vi "L Arm Initial Position.vi"(0 "Cluster":T1={"Axis"={"X"=0.0, "Y"=0.0, "Z"=0.0}, "Arm"=refnum, "EJC"=refnum, "Shoulder Angle"=0.0, "Shoulder Axis"={"X"=-1.0, "Y"=0.0, "Z"=0.0}, "Elbow Angle"=0.0, "Elbow Axis"={"X"=0.0, "Y"=-1.0, "Z"=0.0}}) -> (1 "Scene.Object Out":refnum<vi>, 3 "Scene.Object Out 3":refnum<vi>)   [LabVIEW 2010]
uses:
  <vilib>/picture/3D Picture Control/NI_3D Picture Control.lvlib
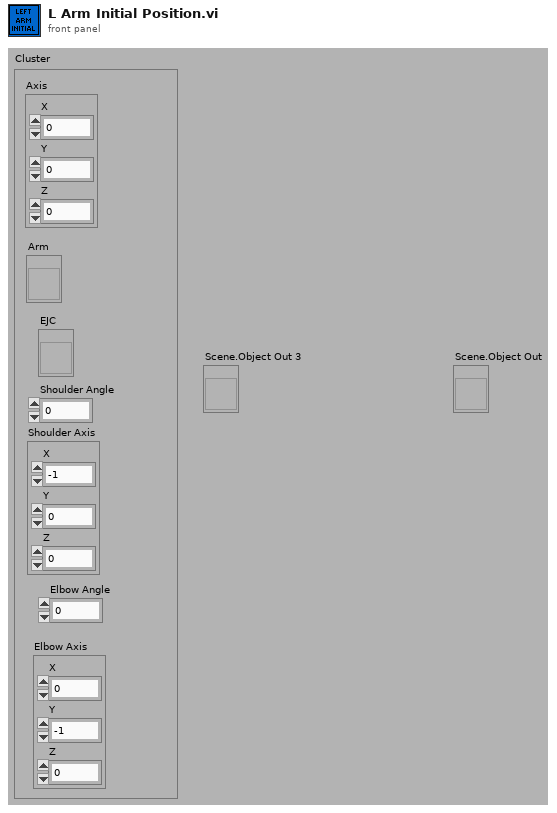
[diagram p1: front panel]
types:
  T1 = cluster{"Axis":cluster{"X":sgl, "Y":sgl, "Z":sgl}, "Arm":refnum<vi>, "EJC":refnum<vi>, "Shoulder Angle":dbl, "Shoulder Axis":cluster{"X":sgl, "Y":sgl, "Z":sgl}, "Elbow Angle":dbl, "Elbow Axis":cluster{"X":sgl, "Y":sgl, "Z":sgl}}
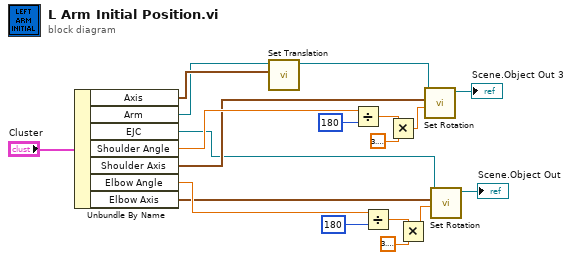
[diagram p0: block diagram]
diagram:
  n1 = Unbundle By Name("Cluster") -> ("Axis"=w4:cluster{"X":sgl, "Y":sgl, "Z":sgl}, "Arm"=w3:refnum<vi>, "EJC"=w2:refnum<vi>, "Shoulder Angle"=w8:dbl, "Shoulder Axis"=w7:cluster{"X":sgl, "Y":sgl, "Z":sgl}, "Elbow Angle"=w6:dbl, "Elbow Axis"=w5:cluster{"X":sgl, "Y":sgl, "Z":sgl})
  n2 = call <vilib>:"Set Translation.vi"("Translation"=w4, "Scene Object"=w3) -> ("Translated Object"=w1:refnum<vi>)  [unwired: 8 in, 1 out]
  n3 = Divide(x=w8, y=180) -> (x/y=w16:dbl)
  n4 = Divide(x=w6, y=180) -> (x/y=w11:dbl)
  n5 = Multiply(x=w16, y=3.141592653589793) -> (x*y=w14:dbl)
  n6 = Multiply(x=w11, y=3.141592653589793) -> (x*y=w13:dbl)
  n7 = call <vilib>:"Set Rotation.vi"("Angle"=w14, "Axis"=w7, "Scene Object"=w1) -> ("Rotated Scene Object"=→"Scene.Object Out 3":refnum<vi>)  [unwired: 7 in, 1 out]
  n8 = call <vilib>:"Set Rotation.vi"("Angle"=w13, "Axis"=w5, "Scene Object"=w2) -> ("Rotated Scene Object"=→"Scene.Object Out":refnum<vi>)  [unwired: 7 in, 1 out]
